vi "Run_FFID_Bkgnd.vi"(3 "Simulated Time":timestamp, 4 "Run Now?":bool, 5 "Simulate/Run":T2) -> (0 "Error Messages":string, 2 "Status":T1)   [LabVIEW 2011]
uses:
  Controls/User_Specific_mode.ctl
  Gen Trav/Multi_Run_Status.ctl
  Controls/Multi_run_mode.ctl
  Globals/Trav_pos_global.vi
  Globals/Extra_Commands_Global.vi
  Globals/Constants_global.vi
panel:
  in  "User Specific":refnum<vi>
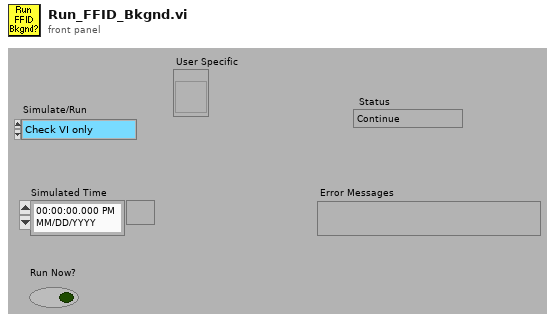
[diagram p1: front panel]
types:
  T1 = typedef "Multi_Run_Status.ctl" = enum16{"Continue", "Jump to Next Point", "Jump to Next Row", "Jump To Fall Back", "Terminate Run"}
  T2 = typedef "User_Specific_mode.ctl" = enum16{"Check VI only", "Run VI"}
  T3 = typedef "Multi_run_mode.ctl" = enum16{"Move Traverse Only", "Set Tunnel Speed Only", "Set Source Only", "Set Measurement Conditions", "Single Measurement", "Vertical Profile", "Lateral Profile", "Longitudinal Profile", "Explore Volume", "Multi-Axis Profile", "Auto Calibrate", "Meas Fast FID Bkgnd", "Check Beam Power", "Scanning Valve Measurement", "Run VI Named:", "Set ADAM Ch", "Wait (minutes)", "Send Message", "Synchronize With:", "Fall Back to this Row", "Turn Off Row Repeating", "Blank Row", "Traverse 3D Volume"}
  T4 = typedef "Traverse_cluster.ctl" = cluster{"Start X":dbl, "Start Y":dbl, "Start Z":dbl, "End X":dbl, "End Y":dbl, "End Z":dbl, "No. of pts.":i32, "Spacing":T5, "Filename":path, "Tunnel Speed":dbl, "Averaging time (min)":dbl, "Extra Commands":string, "Specific Arguments":string, "Emission Rate (l/min)":dbl, "Trace Gas Concentration (%)":dbl, "Density Ratio":string, "Comments":string, "Row No":i32, "Row Type Selector":T3, "Completion time":string, "Row Duration (mins)":dbl, "No. of Valid pts.":i32, "Meas Setup File":string}
  T5 = typedef "Spacing.ctl" = enum16{"Linear", "Log", "Gauss", "Specified", "N/A"}
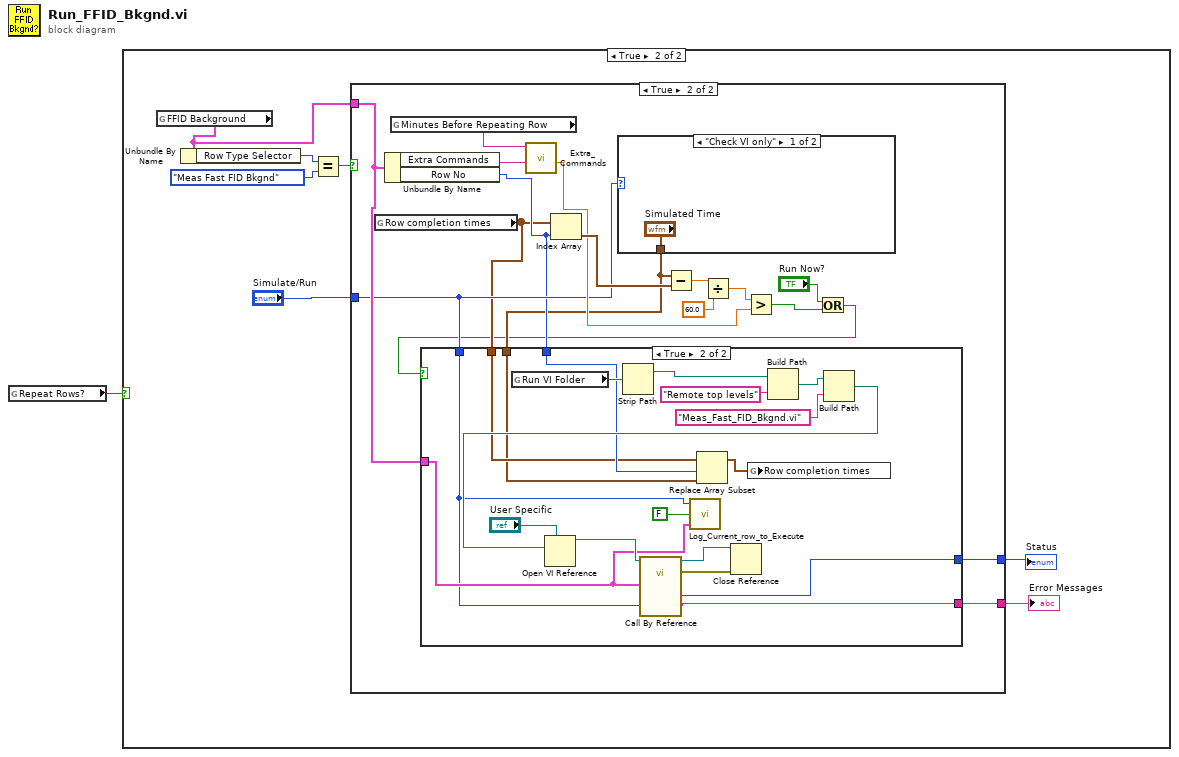
[diagram p0: block diagram]
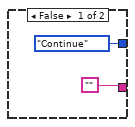
[diagram p3: hidden frame]
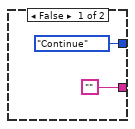
[diagram p4: hidden frame]
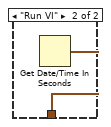
[diagram p5: hidden frame]
diagram:
  n1 = global read "Trav_pos_global.vi" "Repeat Rows?"() -> (w1:bool)
  n2 = case shown="True" w1 {
    frame False {
    }
    frame True {
      n3 = global read "Trav_pos_global.vi" "FFID Background"() -> (w6:T4)
      n4 = Unbundle By Name(w6) -> ("Row Type Selector"=w7:T3)
      n5 = Equal?(x=w7, y=Multi_run_mode."Meas Fast FID Bkgnd" ("Row Type Selector")) -> (x = y?=w5:bool)
      n6 = case shown="True" w5 {
        tunnel: w6 -> [_ w20]
        tunnel: "Simulate/Run" -> [_ w19]
        tunnel: [Multi_Run_Status."Continue" ("Status") w18] -> w3
        tunnel: ["" w17] -> w2
        frame False {
        }
        frame True {
          n7 = global read "Trav_pos_global.vi" "Row completion times"() -> (w15:timestamp[])
          n8 = Unbundle By Name(w20) -> ("Extra Commands"=w27:string, "Row No"=w16:i32)
          n9 = global read "Extra_Commands_Global.vi" "Minutes Before Repeating Row"() -> (w26:string)
          n10 = call "Extra_Commands.vi"("String to Search"=w27, "Command"=w26) -> ("Numeric Value"=w21:dbl)  [unwired: 1 in, 4 out]
          n11 = Index Array(array=w15, index=w16) -> (element=w25:timestamp)
          n12 = case shown="\"Check VI only\"" w19 {
            tunnel: ["Simulated Time" w50] -> w14
            frame "Check VI only" {
            }
            frame "Run VI" {
              n13 = Get Date/Time In Seconds() -> (seconds since 1Jan1904=w50:timestamp)
            }
          }
          n14 = Subtract(x=w14, y=w25) -> (x-y=w24:dbl)
          n15 = Divide(x=w24, y=60.0) -> (x/y=w23:dbl)
          n16 = Greater?(x=w23, y=w21) -> (0:w12:bool)
          n17 = Or(x="Run Now?", y=w12) -> (x .or. y?=w11:bool)
          n18 = case shown="True" w11 {
            tunnel: w20 -> [_ w31]
            tunnel: w19 -> [_ w30]
            tunnel: [Multi_Run_Status."Continue" ("Status") w38] -> w18
            tunnel: ["" w37] -> w17
            tunnel: w16 -> [_ w36]
            tunnel: w15 -> [_ w35]
            tunnel: w14 -> [_ w34]
            frame False {
            }
            frame True {
              n19 = global read "Constants_global.vi" "Run VI Folder"() -> (w48:path)
              n20 = Strip Path(path=w48) -> (stripped path=w47:path)  [unwired: 1 out]
              n21 = call "Log_Current_row_to_Execute.vi"("Simulate/Run"=w30, "Start of Multi Run Prog"=FALSE, "Traverse line in"=w31) -> ()  [unwired: 2 in, 5 out]
              n22 = Replace Array Subset(array=w35, new element=w34, index=w36) -> (w33:timestamp[])
              n23 = global write "Trav_pos_global.vi" "Row completion times"(w33) -> ()
              n24 = Build Path(base path=w47, name or relative path="Remote top levels") -> (appended path=w44:path)
              n25 = Build Path(base path=w44, name or relative path="Meas_Fast_FID_Bkgnd.vi") -> (appended path=w40:path)
              n26 = Open VI Reference(type specifier VI Refnum (for type only)="User Specific", vi path=w40) -> (vi reference=w39:refnum<vi>)  [unwired: 2 in, 3 out]
              n27 = call-by-ref "?"(reference=w39, "Mode"=w30, "Traverse line In"=w31) -> (reference out=w42:refnum<vi>, error out=w43:errorcluster, "Error Message"=w37:string, "Status"=w38:T1)  [unwired: 2 in, 1 out]
              n28 = Close Reference(reference=w42, error in (no error)=w43) -> ()  [unwired: 1 out]
            }
          }
        }
      }
      "Status" <- w3
      "Error Messages" <- w2
    }
  }
